vi "[Global] Image Overlay.vi"() -> ()   [LabVIEW 2019]
panel:
  out "ImageOverlayArray":T1[](array[plugin-control])
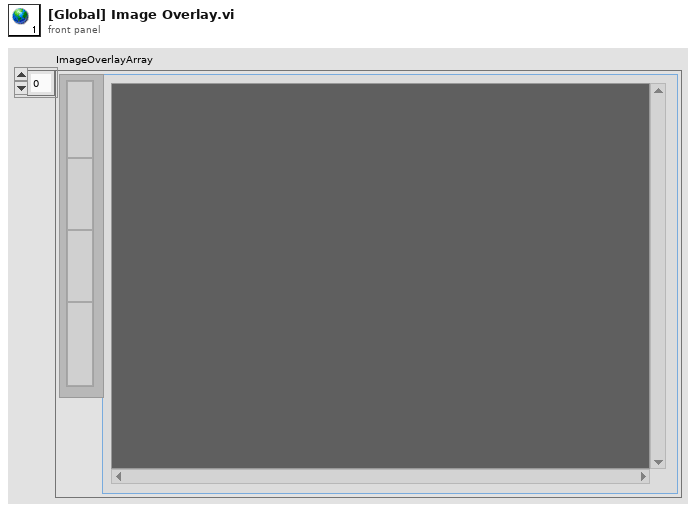
[diagram p1: front panel]
types:
  T1 = typedef "IMAQ Image.ctl" = refnum<image>
diagram:
